vi "GetExecutingJobInformation.vi"(0 "error in (no error)":errorcluster, 9 "HighSpeedEServer":refnum<k24>) -> (4 "error out":errorcluster, 6 "Name":string, 8 "Line":i32, 10 "Step":i32, 15 "SpeedOverride":i32)   [LabVIEW 2023, in "UnderAutomation.Yaskawa.lvlib"]
uses:
  UnderAutomation.Yaskawa.lvlib
  C:/Users/fg/Documents/Yaskawa.vi/LabVIEW_2024/UnderAutomation.Yaskawa/lib/UnderAutomation.Yaskawa.dll
  LabVIEW_2024/UnderAutomation.Yaskawa/lib/UnderAutomation.Yaskawa.dll
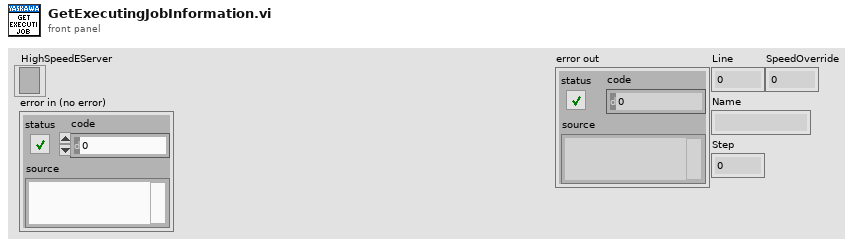
[diagram p1: front panel]
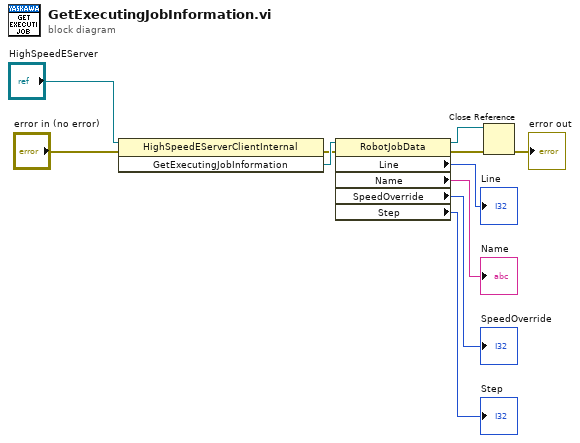
[diagram p0: block diagram]
diagram:
  n1 = invoke class="HighSpeedEServerClientInternal" method="GetExecutingJobInformation"(reference="HighSpeedEServer", error in="error in (no error)") -> (error out=w4:errorcluster, "GetExecutingJobInformation"=w9:refnum<k24>)  [unwired: 1 in, 1 out]
  n2 = property class="RobotJobData"(reference=w9, error in=w4) -> (reference out=w1:refnum<k24>, error out=w3:errorcluster, "Line"=→"Line":i32, "Name"=→"Name":string, "SpeedOverride"=→"SpeedOverride":i32, "Step"=→"Step":i32)
  n3 = Close Reference(reference=w1, error in (no error)=w3) -> (error out=→"error out":errorcluster)
